vi "FlakyDelegate.vi"(4 "Relayed event":refnum<user-event>, 5 "Event Data":cluster{"Event to be relayed":i32}, 6 "User Event Ref":refnum<user-event>, 7 "Event Common Data":T2 {"Event Source" items=["LabVIEW UI"=0, "ActiveX"=1, "User Event"=25]}) -> ()   [LabVIEW 2012]
uses:
  <vilib>/event_ctls.llb/eventsource.ctl
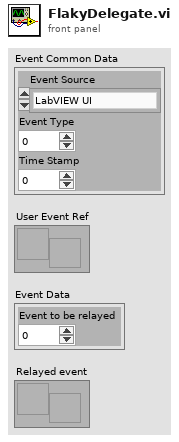
[diagram p1: front panel]
types:
  T1 = typedef "eventsource.ctl" = u32
  T2 = cluster{"Event Source":T1, "Event Type":u32, "Time Stamp":u32}
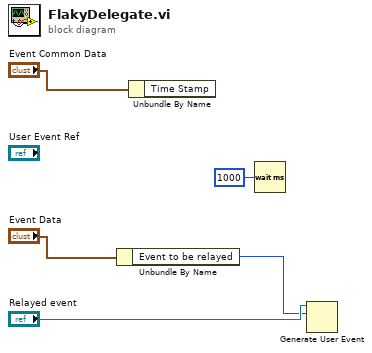
[diagram p0: block diagram]
diagram:
  n1 = Unbundle By Name("Event Data") -> ("Event to be relayed"=w3:i32)
  n2 = Unbundle By Name("Event Common Data") -> ()  [unwired: 1 out]
  n3 = Wait (ms)(milliseconds to wait=u32 1000) -> ()  [unwired: 1 out]
  n4 = Generate User Event(user event="Relayed event", event data cluster=w3) -> ()  [unwired: 1 in, 2 out]
